vi "Input Variants.vi"(0 "Numeric Variant":variant=variant(dbl 4.0) caption="Numeric Variant Caption", 1 "Boolean Array Variant":variant=variant(bool[] [TRUE, FALSE, TRUE, FALSE]), 5 "Boolean Variant":variant=variant(bool TRUE), 9 "String Variant":variant=variant(string "hello"), 11 "Numeric Array Variant":variant=variant(u8[] [1, 2, 3]), 12 "String Array Variant":variant=variant(string[] ["str1", "str2", "str3"])) -> (3 "Boolean Array":bool[](array[boolean])=[TRUE, FALSE, TRUE, FALSE], 4 "Numeric":u32=4, 6 "Boolean":bool=TRUE, 8 "error out":errorcluster, 10 "String":string="hello", 14 "String Array":string[](array[string])=["str1", "str2", "str3"], 15 "Numeric Array":dbl[](array[numeric])=[1.0, 2.0, 3.0] format="%0.2f")   [LabVIEW 2011]
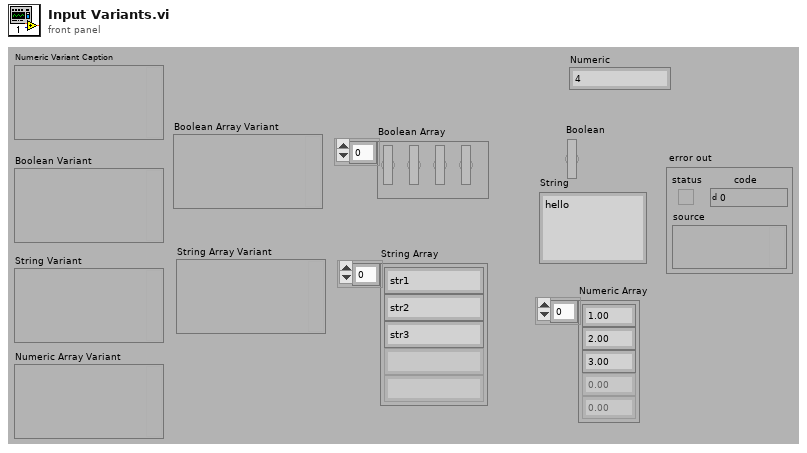
[diagram p1: front panel]
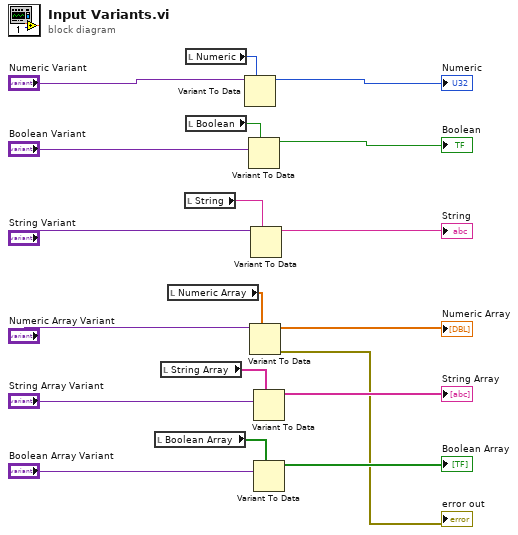
[diagram p0: block diagram]
diagram:
  n1 = local read "Boolean Array"() -> (w5:bool[])
  n2 = local read "String Array"() -> (w8:string[])
  n3 = local read "Numeric Array"() -> (w11:dbl[])
  n4 = local read "String"() -> (w14:string)
  n5 = local read "Numeric"() -> (w18:u32)
  n6 = local read "Boolean"() -> (w17:bool)
  n7 = Variant To Data(type=w18, Variant="Numeric Variant") -> (data=→"Numeric":u32)  [unwired: 1 in, 1 out]
  n8 = Variant To Data(type=w17, Variant="Boolean Variant") -> (data=→"Boolean":bool)  [unwired: 1 in, 1 out]
  n9 = Variant To Data(type=w11, Variant="Numeric Array Variant") -> (data=→"Numeric Array":dbl[], error out=→"error out":errorcluster)  [unwired: 1 in]
  n10 = Variant To Data(type=w14, Variant="String Variant") -> (data=→"String":string)  [unwired: 1 in, 1 out]
  n11 = Variant To Data(type=w8, Variant="String Array Variant") -> (data=→"String Array":string[])  [unwired: 1 in, 1 out]
  n12 = Variant To Data(type=w5, Variant="Boolean Array Variant") -> (data=→"Boolean Array":bool[])  [unwired: 1 in, 1 out]
